vi "Robot Global Data.vi"() -> ()   [LabVIEW 2013]
doc: "This global VI can contain as many global variables as you need. Place a control on the panel, give it a good name. To read or write to it from a VI, drag the icon to the diagram of that VI. You can also drag from the project. Click on the node to change which global you access. You shouldn't have multiple locations writing to a global or it will cause a race-condition."
uses:
  <vilib>/Rock Robotics/WPI/Camera/WPI_CameraImageSize.ctl
  <vilib>/Rock Robotics/WPI/DriverStation/WPI_DriverStationRobotMode2.ctl
panel:
  in  "HarvClear":bool
  in  "HarvestStart":bool
  in  "HarvSetPoint":dbl[](array[numeric])=[1.0, 2.0, 3.0]
  in  "WinchButPressed":bool
  in  "WinchCase":dbl=1.5
  in  "Sorted Array":string[](array[string])
  in  "ManualControl":bool
  in  "CamFireReady":bool
  out "CamPower":dbl
  in  "CamOutGearPos":dbl=1.5
  in  "CamInGearPos":dbl=1.5
  in  "CamPos":dbl=1.5
  in  "CamFire":bool
  out "Harvester POT":dbl
  out "HarvRoller":dbl
  out "HarvPower":dbl
  in  "HarvPot":dbl
  in  "WinchPower":dbl=0.75
  in  "WinchSetPointArray":dbl[](array[numeric])=[1.0, 2.0, 3.0]
  in  "Winch Pot Location":dbl
  out "Winch Motor Power Out":dbl
  out "Encoder":dbl
  out "Auton Array":dbl[][](array[numeric]) format="%0.3f"
  out "Current File":dbl
  out "Auton Files":string[](array[string])
  out "Number of Auton Files":dbl
  in  "Robot Mode":T1
  in  "LED toggle rate (ms)":u32=20
  in  "image size":T2=enum."320x240"
  in  "Enable Vision":bool
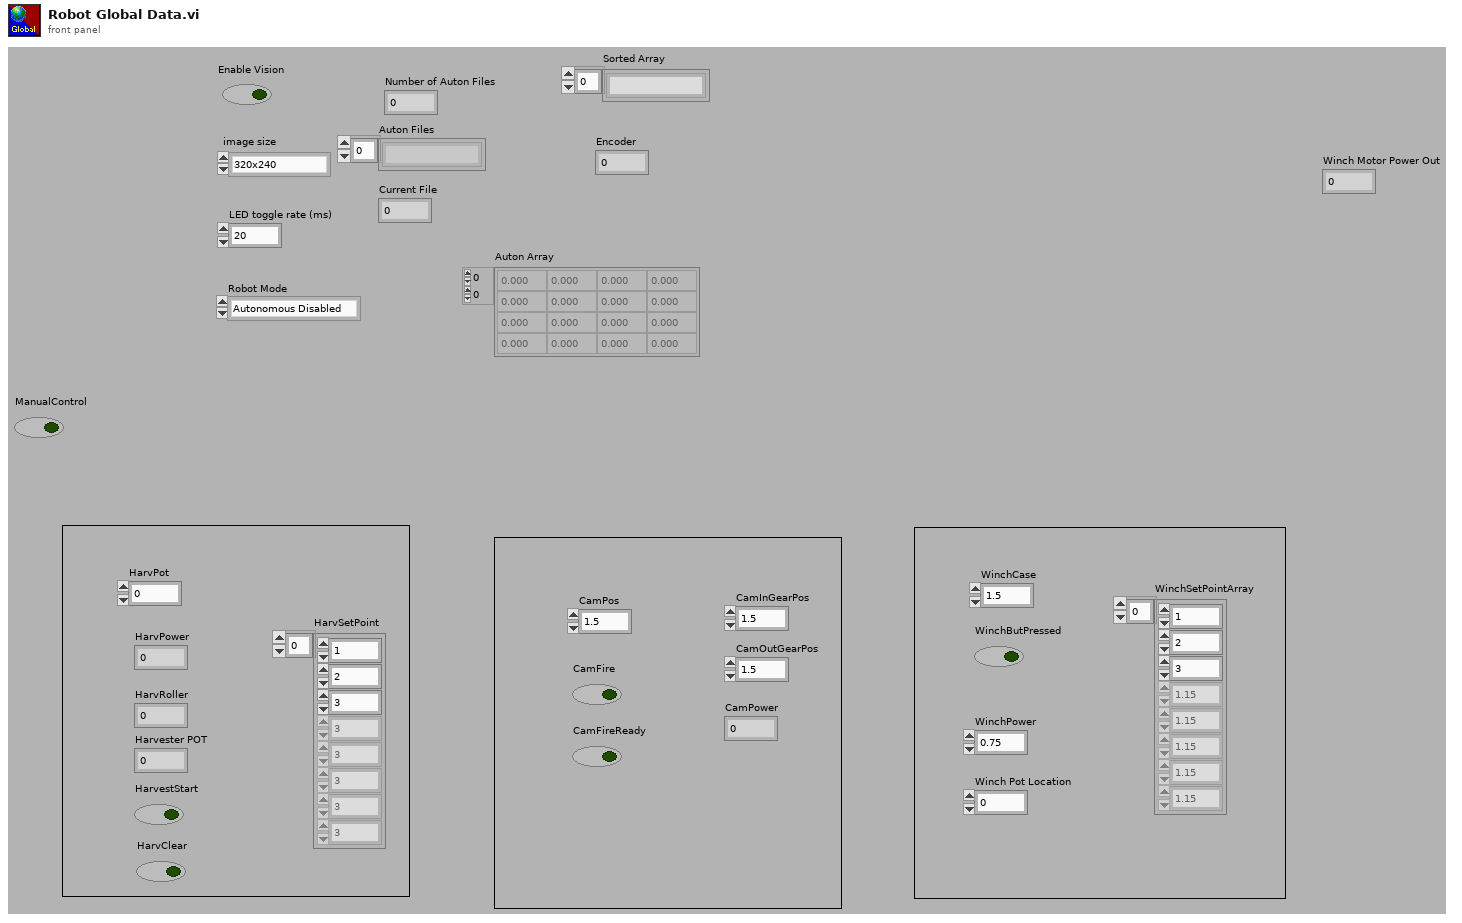
[diagram p1: front panel]
types:
  T1 = typedef "WPI_DriverStationRobotMode2.ctl" = enum16{"Autonomous Disabled", "Autonomous Enabled", "Teleop Disabled", "Teleop Enabled", "Timeout", "Finish", "Test Disabled", "Test Enabled"}
  T2 = typedef "WPI_CameraImageSize.ctl" = enum16{"640x480", "320x240", "160x120"}
diagram:
